vi "Arduino Buffer communication tester.vi"() -> ()   [LabVIEW 2021]
uses:
  <vilib>/Instr/_visa.llb/VISA Configure Serial Port (Instr).vi
panel:
  in  "write buffer":string
  out "read buffer":string
  in  "stop":bool
  in  "VISA resource name":refnum<visa-resource-name>="COM13"
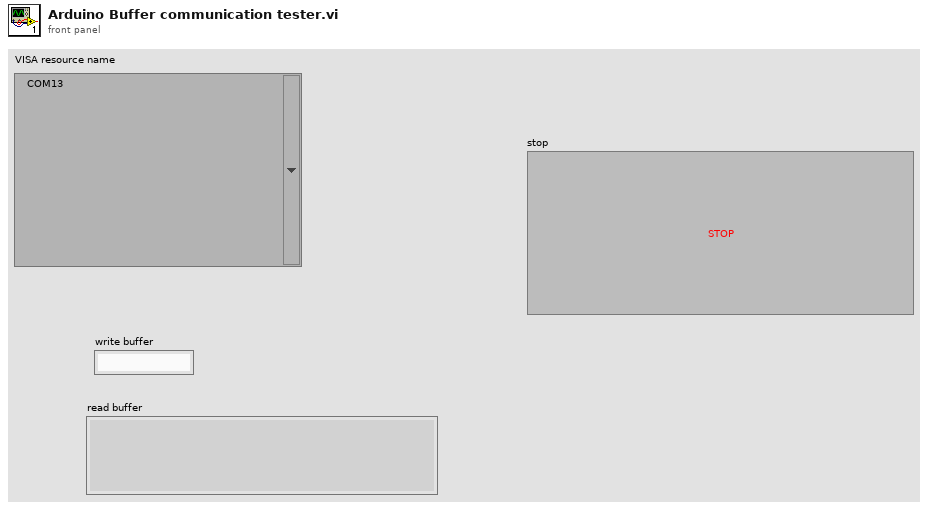
[diagram p1: front panel]
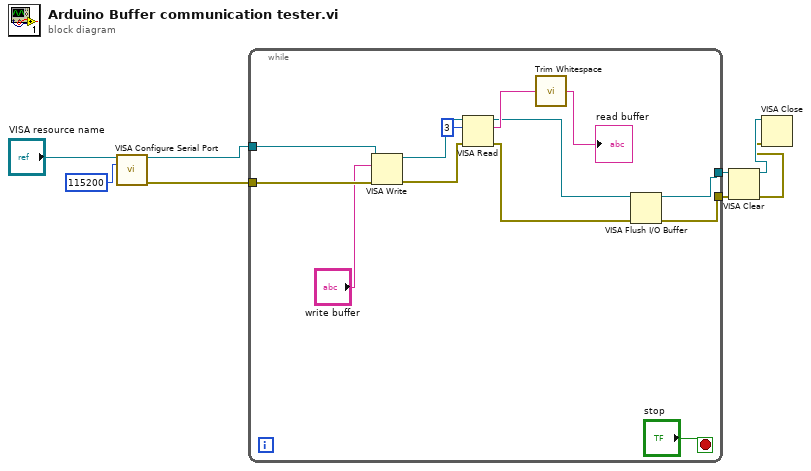
[diagram p0: block diagram]
diagram:
  n1 = call-poly "VISA Configure Serial Port"("VISA resource name"="VISA resource name", "baud rate (9600)"=u32 115200) -> ("VISA resource name out"=w4:refnum<visa-resource-name>, "error out"=w3:errorcluster)  [unwired: 12 in]
  n2 = while {
    tunnel: w4 -> [w17]
    tunnel: w3 -> [w16]
    tunnel: [w12] -> w2
    tunnel: [w11] -> w1
    stop <- "stop" stop-if-true
    n3 = VISA Write(VISA resource name=w17, write buffer="write buffer", error in (no error)=w16) -> (VISA resource name out=w20:refnum<visa-resource-name>, error out=w19:errorcluster)  [unwired: 1 out]
    n4 = VISA Read(VISA resource name=w20, byte count=u32 3, error in (no error)=w19) -> (VISA resource name out=w13:refnum<visa-resource-name>, read buffer=w15:string, error out=w10:errorcluster)  [unwired: 1 out]
    n5 = call <vilib>:"Trim Whitespace.vi"("string"=w15) -> ("trimmed string"=→"read buffer":string)  [unwired: 1 in]
    n6 = VISA Flush I/O Buffer(VISA resource name=w13, error in (no error)=w10) -> (VISA resource name out=w12:refnum<visa-resource-name>, error out=w11:errorcluster)  [unwired: 1 in]
  }
  n7 = VISA Clear(VISA resource name=w2, error in (no error)=w1) -> (VISA resource name out=w8:refnum<visa-resource-name>, error out=w7:errorcluster)
  n8 = VISA Close(VISA resource name=w8, error in (no error)=w7) -> ()  [unwired: 1 out]
